vi "IntegerParityDetector.vi"() -> ()   [LabVIEW 2017]
panel:
  out "Odd?":bool
  in  "Integer":i32
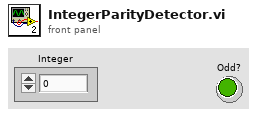
[diagram p1: front panel]
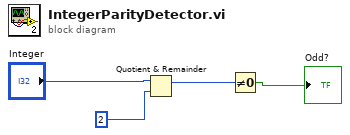
[diagram p0: block diagram]
diagram:
  n1 = Quotient & Remainder(x="Integer", y=2) -> (x-y*floor(x/y)=w2:i32)  [unwired: 1 out]
  n2 = Not Equal To 0?(x=w2) -> (x != 0?=→"Odd?":bool)
